vi "Test Delete Cache.vi"() -> (0 "error out":errorcluster)   [LabVIEW 2020]
doc: "Test <b>Delete Cache</b> VI from public API."
uses:
  src/Path Getter Mock/Path Getter Mock.lvclass
  C:/Users/juanj/Documents/hasbun_wood_engineering/github/Debug-Snapshots-for-LabVIEW/src/IPath Getter/IPath Getter.lvclass
  <userlib>/_OpenG.lib/file/file.llb/File Exists - Scalar__ogtk.vi
  <vilib>/addons/_JKI Toolkits/Caraya/classes/Test/Test.lvclass
  <userlib>/_OpenG.lib/file/file.llb/openg_file.lvlib
  src/Public API.lvlib
  <vilib>/addons/_JKI Toolkits/Caraya/classes/Assert/Assert.lvclass
  C:/Users/juanj/Documents/hasbun_wood_engineering/github/Debug-Snapshots-for-LabVIEW/src/Path Getter Mock/Path Getter Mock.lvclass
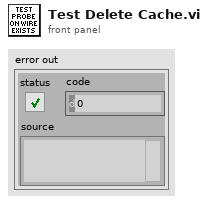
[diagram p1: front panel]
types:
  T1 = enum16{"open", "replace", "create", "open or create", "replace or create", "replace or create with confirmation"}
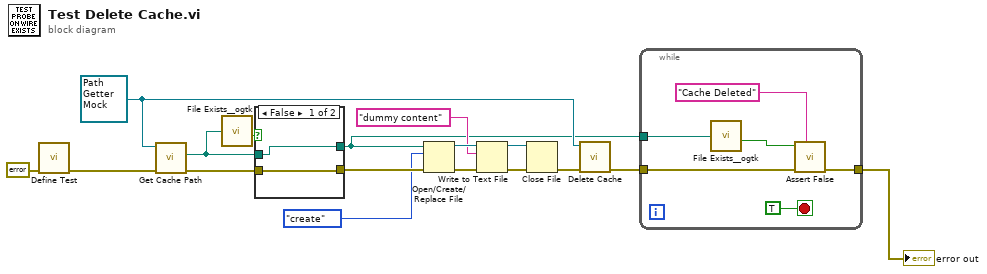
[diagram p0: block diagram]
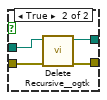
[diagram p2: hidden frame]
diagram:
  w6 = refnum<class "Path Getter Mock.lvclass"> refnum ("Path Getter Mock.lvclass")
  n1 = call <vilib>:"Define Test.vi"("error in (no error)"=errorcluster {"status"=FALSE, "code"=0, "source"=""}) -> ("error out"=w15:errorcluster)  [unwired: 9 in, 1 out]
  n2 = call-dynamic "Get Cache Path.vi"("error in"=w15, "Path Getter Mock in"=w6) -> ("error out"=w16:errorcluster, "Path"=w2:path)  [unwired: 8 in]
  n3 = call-poly <userlib>:"File Exists__ogtk.vi"("file path"=w2) -> ("exists"=w1:bool)  [unwired: 6 in, 1 out]
  n4 = case shown="False" w1 {
    tunnel: w16 -> [w18 w23]
    tunnel: [w18 w22] -> w14
    tunnel: [w19 w21] -> w4
    tunnel: w2 -> [w19 w20]
    frame False {
    }
    frame True {
      n5 = call <userlib>:"Delete Recursive__ogtk.vi"("error in (no error)"=w23, "Path"=w20) -> ("error out"=w22:errorcluster, "dup Path"=w21:path)  [unwired: 8 in]
    }
  }
  n6 = Open/Create/Replace File(file path (use dialog)=w4, error in=w14, operation (0:open)=T1."create") -> (refnum out=w11:refnum<file>, error out=w12:errorcluster)  [unwired: 3 in, 1 out]
  n7 = Write to Text File(file (use dialog)=w11, text="dummy content", error in=w12) -> (refnum out=w9:refnum<file>, error out=w8:errorcluster)  [unwired: 1 in, 1 out]
  n8 = Close File(refnum=w9, error in=w8) -> (error out=w7:errorcluster)  [unwired: 1 out]
  n9 = call "Delete Cache.vi"("error in"=w7, "IPath Getter.lvclass"=w6) -> ("error out"=w5:errorcluster)  [unwired: 9 in]
  n10 = while {
    tunnel: w5 -> [w26]
    tunnel: w4 -> [w28]
    tunnel: [w24] -> w3
    stop <- TRUE stop-if-true
    n11 = call-poly <userlib>:"File Exists__ogtk.vi"("file path"=w28) -> ("exists"=w27:bool)  [unwired: 6 in, 1 out]
    n12 = call <vilib>:"Assert False.vi"("Label"="Cache Deleted", "error in (no error)"=w26, "False?"=w27) -> ("error out"=w24:errorcluster)  [unwired: 7 in, 1 out]
  }
  "error out" <- w3
